vi "PID Intake.vi"(6 "Encoder Overide":bool, 8 "Limit":bool, 9 "Setpoint Intake":dbl, 10 "MotorControlDevRef":T1, 11 "PID Constants":T7={"P Gain"=0.15, "I Gain"=1e-05, "D Gain"=0.0, "F Gain"=0.0, "I Zone"=10.0, "Min Output"=-0.5, "Max Output"=0.3} {"Max Output" min=-1.0 max=1.0 step=0.01; "Min Output" min=-1.0 max=1.0 step=0.01; "I Zone" step=0.01; "F Gain" step=0.01; "D Gain" step=0.01; "I Gain" step=0.01; "P Gain" min=0.0 step=0.01}) -> ()   [LabVIEW 2018]
uses:
  <vilib>/Rock Robotics/WPI/MotorControl/WPI_MotorControlDeviceRef.ctl
  <vilib>/Rock Robotics/WPI/MotorControl/WPI_MotorControlType.ctl
  <vilib>/Rock Robotics/SystemInterfaces/DIO/FPGA_DIOPWMChannel.ctl
  <vilib>/Rock Robotics/WPI/PWM/WPI_PWMDeadband.ctl
  <vilib>/Rock Robotics/SystemInterfaces/DIO/FPGA_DIOChannel.ctl
  <vilib>/Rock Robotics/WPI/ThirdParty/REV Robotics/SPARK MAX/Typedef/Spark MAX Control Type.ctl
  Robot Global Data.vi
panel:
  out "PID Chart":T6(graph)
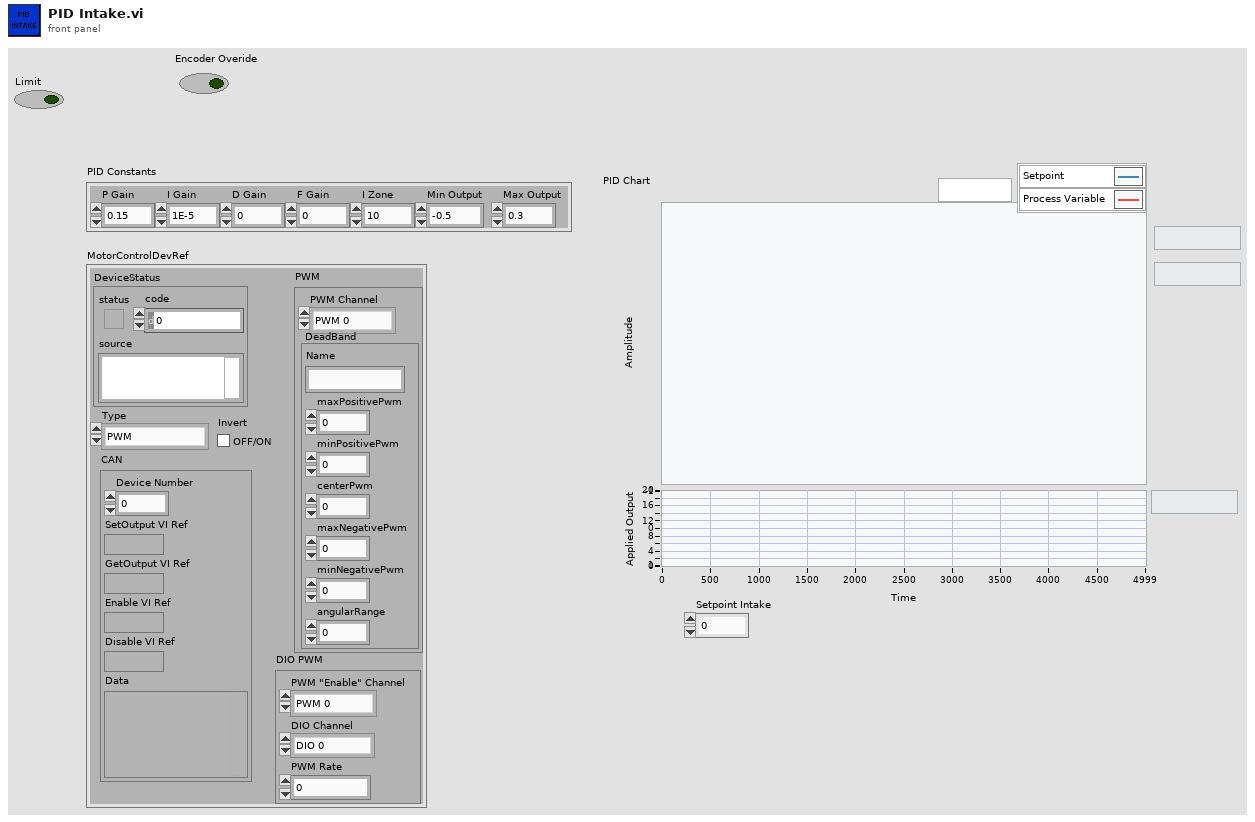
[diagram p1: front panel]
types:
  T1 = typedef "WPI_MotorControlDeviceRef.ctl" = cluster{"DeviceStatus":errorcluster, "Type":T2, "PWM":cluster{"PWM Channel":T3, "DeadBand":T4}, "CAN":cluster{"Device Number":u8, "SetOutput VI Ref":variant, "GetOutput VI Ref":variant, "Enable VI Ref":variant, "Disable VI Ref":variant, "Data":variant}, "Invert":bool, "DIO PWM":cluster{"PWM \"Enable\" Channel":T3, "DIOChannel":T5, "PWM Rate":dbl}}
  T2 = typedef "WPI_MotorControlType.ctl" = enum16{"PWM", "CAN", "DIO PWM"}
  T3 = typedef "FPGA_DIOPWMChannel.ctl" = enum8{"PWM 0", "PWM 1", "PWM 2", "PWM 3", "PWM 4", "PWM 5", "PWM 6", "PWM 7", "PWM 8", "PWM 9", "PWM MXP 0", "PWM MXP 1", "PWM MXP 2", "PWM MXP 3", "PWM MXP 4", "PWM MXP 5", "PWM MXP 6", "PWM MXP 7", "PWM MXP 8", "PWM MXP 9", "Invalid"}
  T4 = typedef "WPI_PWMDeadband.ctl" = cluster{"Name":string, "maxPositivePwm":i32, "minPositivePwm":i32, "centerPwm":i32, "maxNegativePwm":i32, "minNegativePwm":i32, "angularRange":u16}
  T5 = typedef "FPGA_DIOChannel.ctl" = enum8{"DIO 0", "DIO 1", "DIO 2", "DIO 3", "DIO 4", "DIO 5", "DIO 6", "DIO 7", "DIO 8", "DIO 9", "DIO MXP 0", "DIO MXP 1", "DIO MXP 2", "DIO MXP 3", "DIO MXP 4", "DIO MXP 5", "DIO MXP 6", "DIO MXP 7", "DIO MXP 8", "DIO MXP 9", "DIO MXP 10", "DIO MXP 11", "DIO MXP 12", "DIO MXP 13", "DIO MXP 14", "DIO MXP 15", "SPI Port CS1", "SPI Port CS2", "SPI Port CS3", "SPI Port MISO", "SPI Port MOSI", "Invalid"}
  T6 = cluster{"Sensor Velocity":dbl, "Setpoint":dbl, "Applied Output":dbl}
  T7 = cluster{"P Gain":dbl, "I Gain":dbl, "D Gain":dbl, "F Gain":dbl, "I Zone":dbl, "Min Output":dbl, "Max Output":dbl}
  T8 = typedef "Spark MAX Status 0 Frame.ctl" = cluster{"Applied Output":dbl, "Faults":T9, "Sticky Faults":T9, "Rsvd":u8, "Status 0 Flags":T10, "Timestamp":u32}
  T9 = typedef "Spark MAX Faults.ctl" = cluster{"Hard Limit Rev":bool, "Hard Limit Fwd":bool, "Soft Limit Fwd":bool, "Soft Limit Rev":bool, "Other Fault":bool, "DRV Fault":bool, "Has Reset?":bool, "CAN RX":bool, "CAN TX":bool, "EEPROM CRC":bool, "Stall":bool, "Sensor Fault":bool, "Motor Type Fault":bool, "IWDT Reset":bool, "Over Current":bool, "Brownout":bool}
  T10 = typedef "Spark MAX Status 0 Flags.ctl" = cluster{"Invert/Brake":bool, "Is Follower":bool}
  T11 = typedef "Spark MAX Control Type.ctl" = enum16{"Percent VBus", "Voltage", "Velocity", "Position", "Smart Motion", "Current", "Smart Velocity"}
  T12 = cluster{"Sensor Position":dbl, "Setpoint Intake":dbl, "Applied Output":dbl}
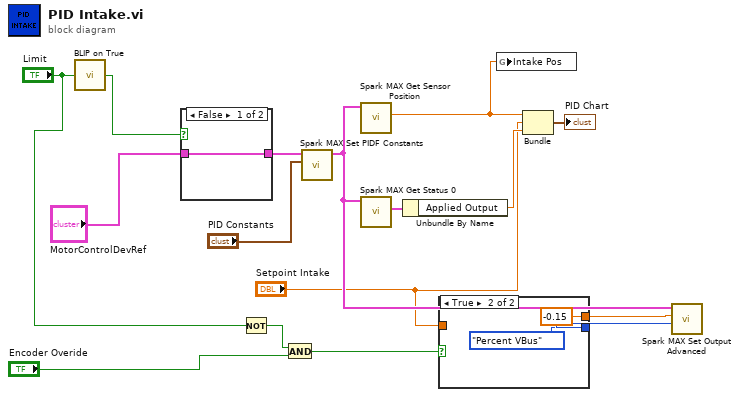
[diagram p0: block diagram]
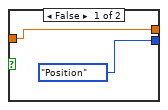
[diagram p2: hidden frame]
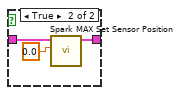
[diagram p3: hidden frame]
diagram:
  n1 = call "BLIP on True.vi"("Boolean Input"="Limit") -> ("Blip on True"=w1:bool)
  n2 = case shown="False" w1 {
    tunnel: "MotorControlDevRef" -> [w17 w20]
    tunnel: [w17 w19] -> w9
    frame False {
    }
    frame True {
      n3 = call <vilib>:"Spark MAX Set Sensor Position.vi"("Position"=0.0, "MotorControlDeviceRef"=w20) -> ("MotorControlDeviceRef"=w19:T1)  [unwired: 8 in, 1 out]
    }
  }
  n4 = Not(x="Limit") -> (.not. x?=w5:bool)
  n5 = And(x=w5, y="Encoder Overide") -> (x .and. y?=w6:bool)
  n6 = call <vilib>:"Spark MAX Set PIDF Constants.vi"("PID Constants"="PID Constants", "MotorControlDeviceRef"=w9) -> ("MotorControlDeviceRef"=w16:T1)  [unwired: 8 in, 1 out]
  n7 = call <vilib>:"Spark MAX Get Sensor Position.vi"("MotorControlDevRef in"=w16) -> ("Sensor Position"=w3:dbl)  [unwired: 7 in, 3 out]
  n8 = call <vilib>:"Spark MAX Get Status 0.vi"("MotorControlDevRef"=w16) -> ("Status 0"=w13:T8)  [unwired: 7 in, 3 out]
  n9 = Unbundle By Name(w13) -> ("Applied Output"=w12:dbl)
  n10 = case shown="True" w6 {
    tunnel: [Spark_MAX_Control_Type."Position" ("Control Mode") Spark_MAX_Control_Type."Percent VBus" ("Control Mode")] -> w11
    tunnel: [w21 -0.15 ("Setpoint Intake")] -> w7
    tunnel: "Setpoint Intake" -> [w21 _]
    frame False {
    }
    frame True {
    }
  }
  n11 = global write "Robot Global Data.vi" "Intake Pos"(w3) -> ()
  n12 = Bundle("Sensor Position"=w3, "Setpoint Intake"="Setpoint Intake", "Applied Output"=w12) -> (→"PID Chart":T12)  [unwired: 1 in]
  n13 = call <vilib>:"Spark MAX Set Output Advanced.vi"("Control Mode"=w11, "Setpoint"=w7, "MotorControlDevRef"=w16) -> ()  [unwired: 7 in, 2 out]
